vi "Create RxTx.vi"(8 "error in (no error)":errorcluster, 11 "Channel GUI in":refnum<class "Channel GUI.lvclass">) -> (0 "error out":errorcluster, 3 "Channel GUI out":refnum<class "Channel GUI.lvclass">)   [LabVIEW 2018, in "Channel GUI.lvclass"]
uses:
  Channel GUI.lvclass
  Channel GUI.lvclass/Channel GUI.ctl
  RxTx/RxTx.lvclass
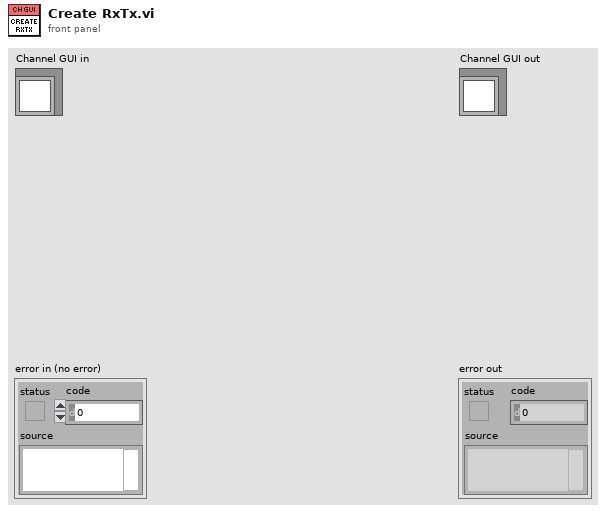
[diagram p1: front panel]
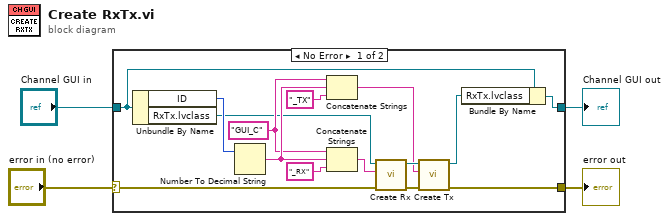
[diagram p0: block diagram]
diagram:
  n1 = case shown="No Error" "error in (no error)" {
    selector: "error in (no error)" -> [w12 w21]
    tunnel: [w9 w21] -> w2
    tunnel: [w18 w20] -> w1
    tunnel: "Channel GUI in" -> [w19 w20]
    frame No Error {
      w13 = "GUI_C"
      n2 = Unbundle By Name(w19) -> ("ID"=w14:u8, "RxTx.lvclass"=w11:refnum<class "RxTx.lvclass">)
      n3 = Number To Decimal String(number=w14) -> (decimal integer string=w15:string)  [unwired: 1 in]
      n4 = Concatenate Strings(w13, w15, "_TX") -> (w5:string)
      n5 = Concatenate Strings(w13, w15, "_RX") -> (w10:string)
      n6 = call "Create Rx.vi"("error in (no error)"=w12, "Reader Name"=w10, "RxTx in"=w11) -> ("error out"=w6:errorcluster, "RxTx out"=w7:refnum<class "RxTx.lvclass">)  [unwired: 7 in]
      n7 = call "Create Tx.vi"("error in (no error)"=w6, "Writer Name"=w5, "RxTx in"=w7) -> ("error out"=w9:errorcluster, "RxTx out"=w8:refnum<class "RxTx.lvclass">)  [unwired: 7 in]
      n8 = Bundle By Name(cluster=w19, "RxTx.lvclass"=w8) -> (w18:refnum<class "Channel GUI.lvclass">)
    }
    frame Error {
    }
  }
  "error out" <- w2
  "Channel GUI out" <- w1
